vi "Save Contact.vi"(6 "Command":T1=enum."Set Position", 8 "error in (no error)":errorcluster, 11 "Contact":T2={"ID"=0, "UUID"="", "Name"="", "Iteration"=0, "Posit Array"=[], "Controls"={"throttle"=0.0, "brake"=0.0, "horn"=0.0, "wait"=0.5}, "DestArray"=[], "SetSpeed"=0.0, "Speed"=0.0, "PathData"={"Path Found?"=FALSE, "Same Line +Dir?"=FALSE, "Path"=[]}}) -> (0 "error out":errorcluster, 3 "dup Contact":T2={"ID"=0, "UUID"="", "Name"="", "Iteration"=0, "Posit Array"=[], "Controls"={"throttle"=0.0, "brake"=0.0, "horn"=0.0, "wait"=0.5}, "DestArray"=[], "SetSpeed"=0.0, "Speed"=0.0, "PathData"={"Path Found?"=FALSE, "Same Line +Dir?"=FALSE, "Path"=[]}})   [LabVIEW 2014, in "Contact Data.lvlib"]
doc: "Updates an existing contact or inserts a new contact into the address book data store. Use the ID of an existing contact to update, or an ID of 0 to insert. When inserting, the output cluster will contain the ID of the new contact."
uses:
  Contact Data.lvlib
  Contact.ctl
  Position.ctl
  Controls.ctl
  DestinationCluster.ctl
  DesinationControls.ctl
  PathData.ctl
  Components/PathFinder/Controls/PathControl.ctl
  Command.ctl
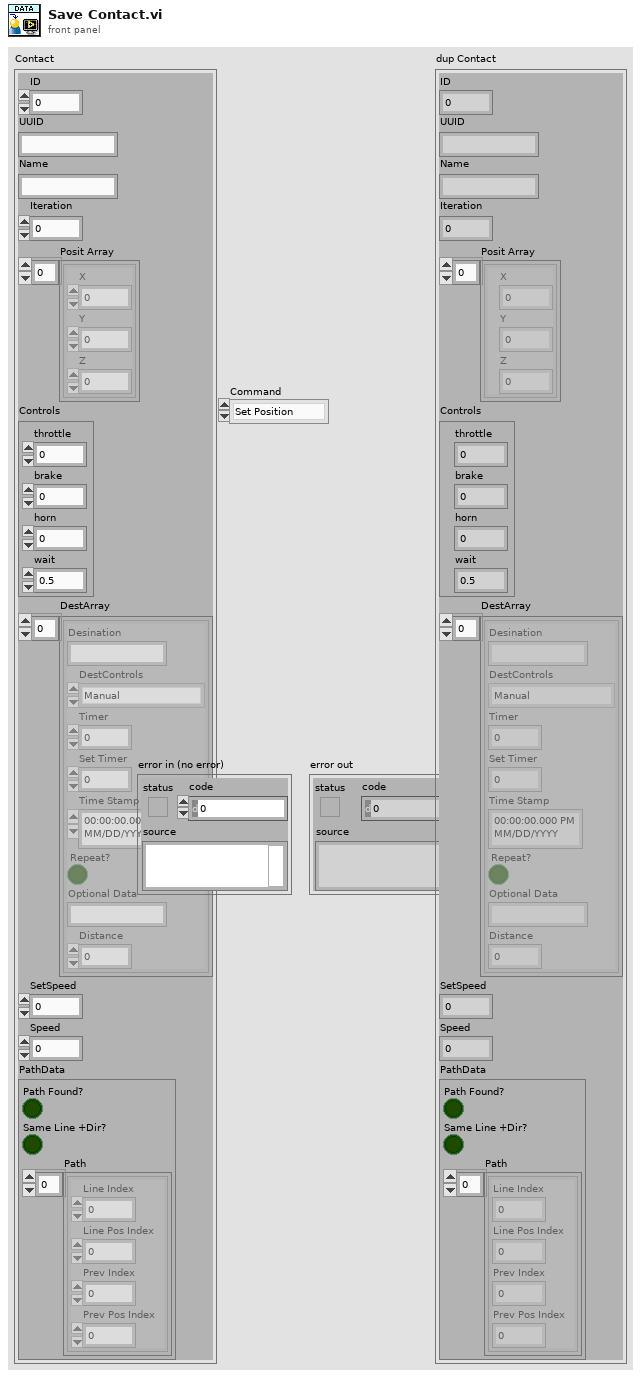
[diagram p1: front panel]
types:
  T1 = typedef "Contact Data.lvlib/Command.ctl" = enum16{"Set All Contacts", "Load", "Save", "Get All Data", "Get Single Data (ID)", "Get Single Data", "Set Position", "Set Destinations", "Set Controls", "Remove Single Data", "Remove UUID Contact", "Set Single ALL", "Is Data Modified", "Import Data"}
  T2 = typedef "Contact Data.lvlib/Contact.ctl" = cluster{"ID":u32, "UUID":string, "Name":string, "Iteration":i32, "Posit Array":T3[], "Controls":T4, "DestArray":T5[], "SetSpeed":dbl, "Speed":dbl, "PathData":T7}
  T3 = typedef "Contact Data.lvlib/Position.ctl" = cluster{"X":dbl, "Y":dbl, "Z":dbl}
  T4 = typedef "Contact Data.lvlib/Controls.ctl" = cluster{"throttle":dbl, "brake":dbl, "horn":dbl, "wait":dbl}
  T5 = typedef "Contact Data.lvlib/DestinationCluster.ctl" = cluster{"Desination":string, "DestControls":T6, "Timer":u32, "Set Timer":u32, "Time Stamp":timestamp, "Repeat?":bool, "Optional Data":string, "Distance":dbl}
  T6 = typedef "Contact Data.lvlib/DesinationControls.ctl" = enum16{"Tracker", "Manual", "Stop", "Station DateTime", "Station Timer", "Maintain"}
  T7 = typedef "Contact Data.lvlib/PathData.ctl" = cluster{"Path Found?":bool, "Same Line +Dir?":bool, "Path":T8[]}
  T8 = typedef "PathControl.ctl" = cluster{"Line Index":i32, "Line Pos Index ":i32, "Prev Index ":i32, "Prev Pos Index":i32}
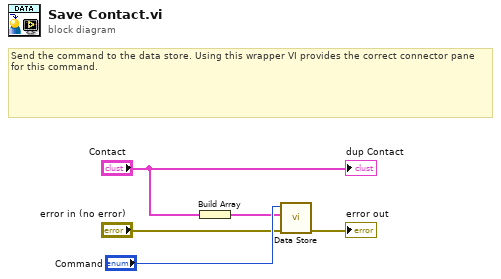
[diagram p0: block diagram]
diagram:
  # "Send the command to the data store. Using this wrapper VI provides the correct connector pane for this command."
  n1 = Build Array("Contact") -> (w1:T2[])
  n2 = call "Data Store.vi"("error in (no error)"="error in (no error)", "Contact in"=w1, "Command"="Command") -> ("error out"=→"error out":errorcluster)  [unwired: 6 in, 2 out]
  "dup Contact" <- "Contact"
